vi "TCPIPClienteTeste.vi"() -> ()   [LabVIEW 2012]
uses:
  Setup File/Setup File.lvclass
  RxTXCamera/RxTxCamera.lvclass
  CCDCamera/CCDCamera.lvclass
  CCDCamera/CCDCamera.lvclass/CCDCamera.ctl
  Construct String Setup Cam/Construct String Setup Cam.lvclass
panel:
  in  "Stop":bool
  in  "Start Acquisition":bool
  in  "CCDCamera.lvclass":refnum<class "CCDCamera.lvclass">
  in  "stop":bool
  out "data out":string
  out "Camera Setup":string
  in  "RxTxCamera in":refnum<class "RxTxCamera.lvclass">
  out "Setup 2":T1
  in  "Setup":T1={"Read Mode"="C", "Acquisition Mode"="A", "Trigger"="B", "Exposure Time"="D", "VShift Speed"="E", "Readout rate"="F", "Pre amp"="G", "Shutter Mode"="H", "Shutter TTL"="I", "Time to open shutter"="J", "Time to close shutter"="K", "Cooler"="L", "Temperature"="M", "Initial Line"="N", "Initial Column"="O", "Final Line"="P", "Final Column"="Q", "Horizontal binning"="R", "Vertical binning"="S"}
  in  "Setup File.lvclass":refnum<class "Setup File.lvclass">
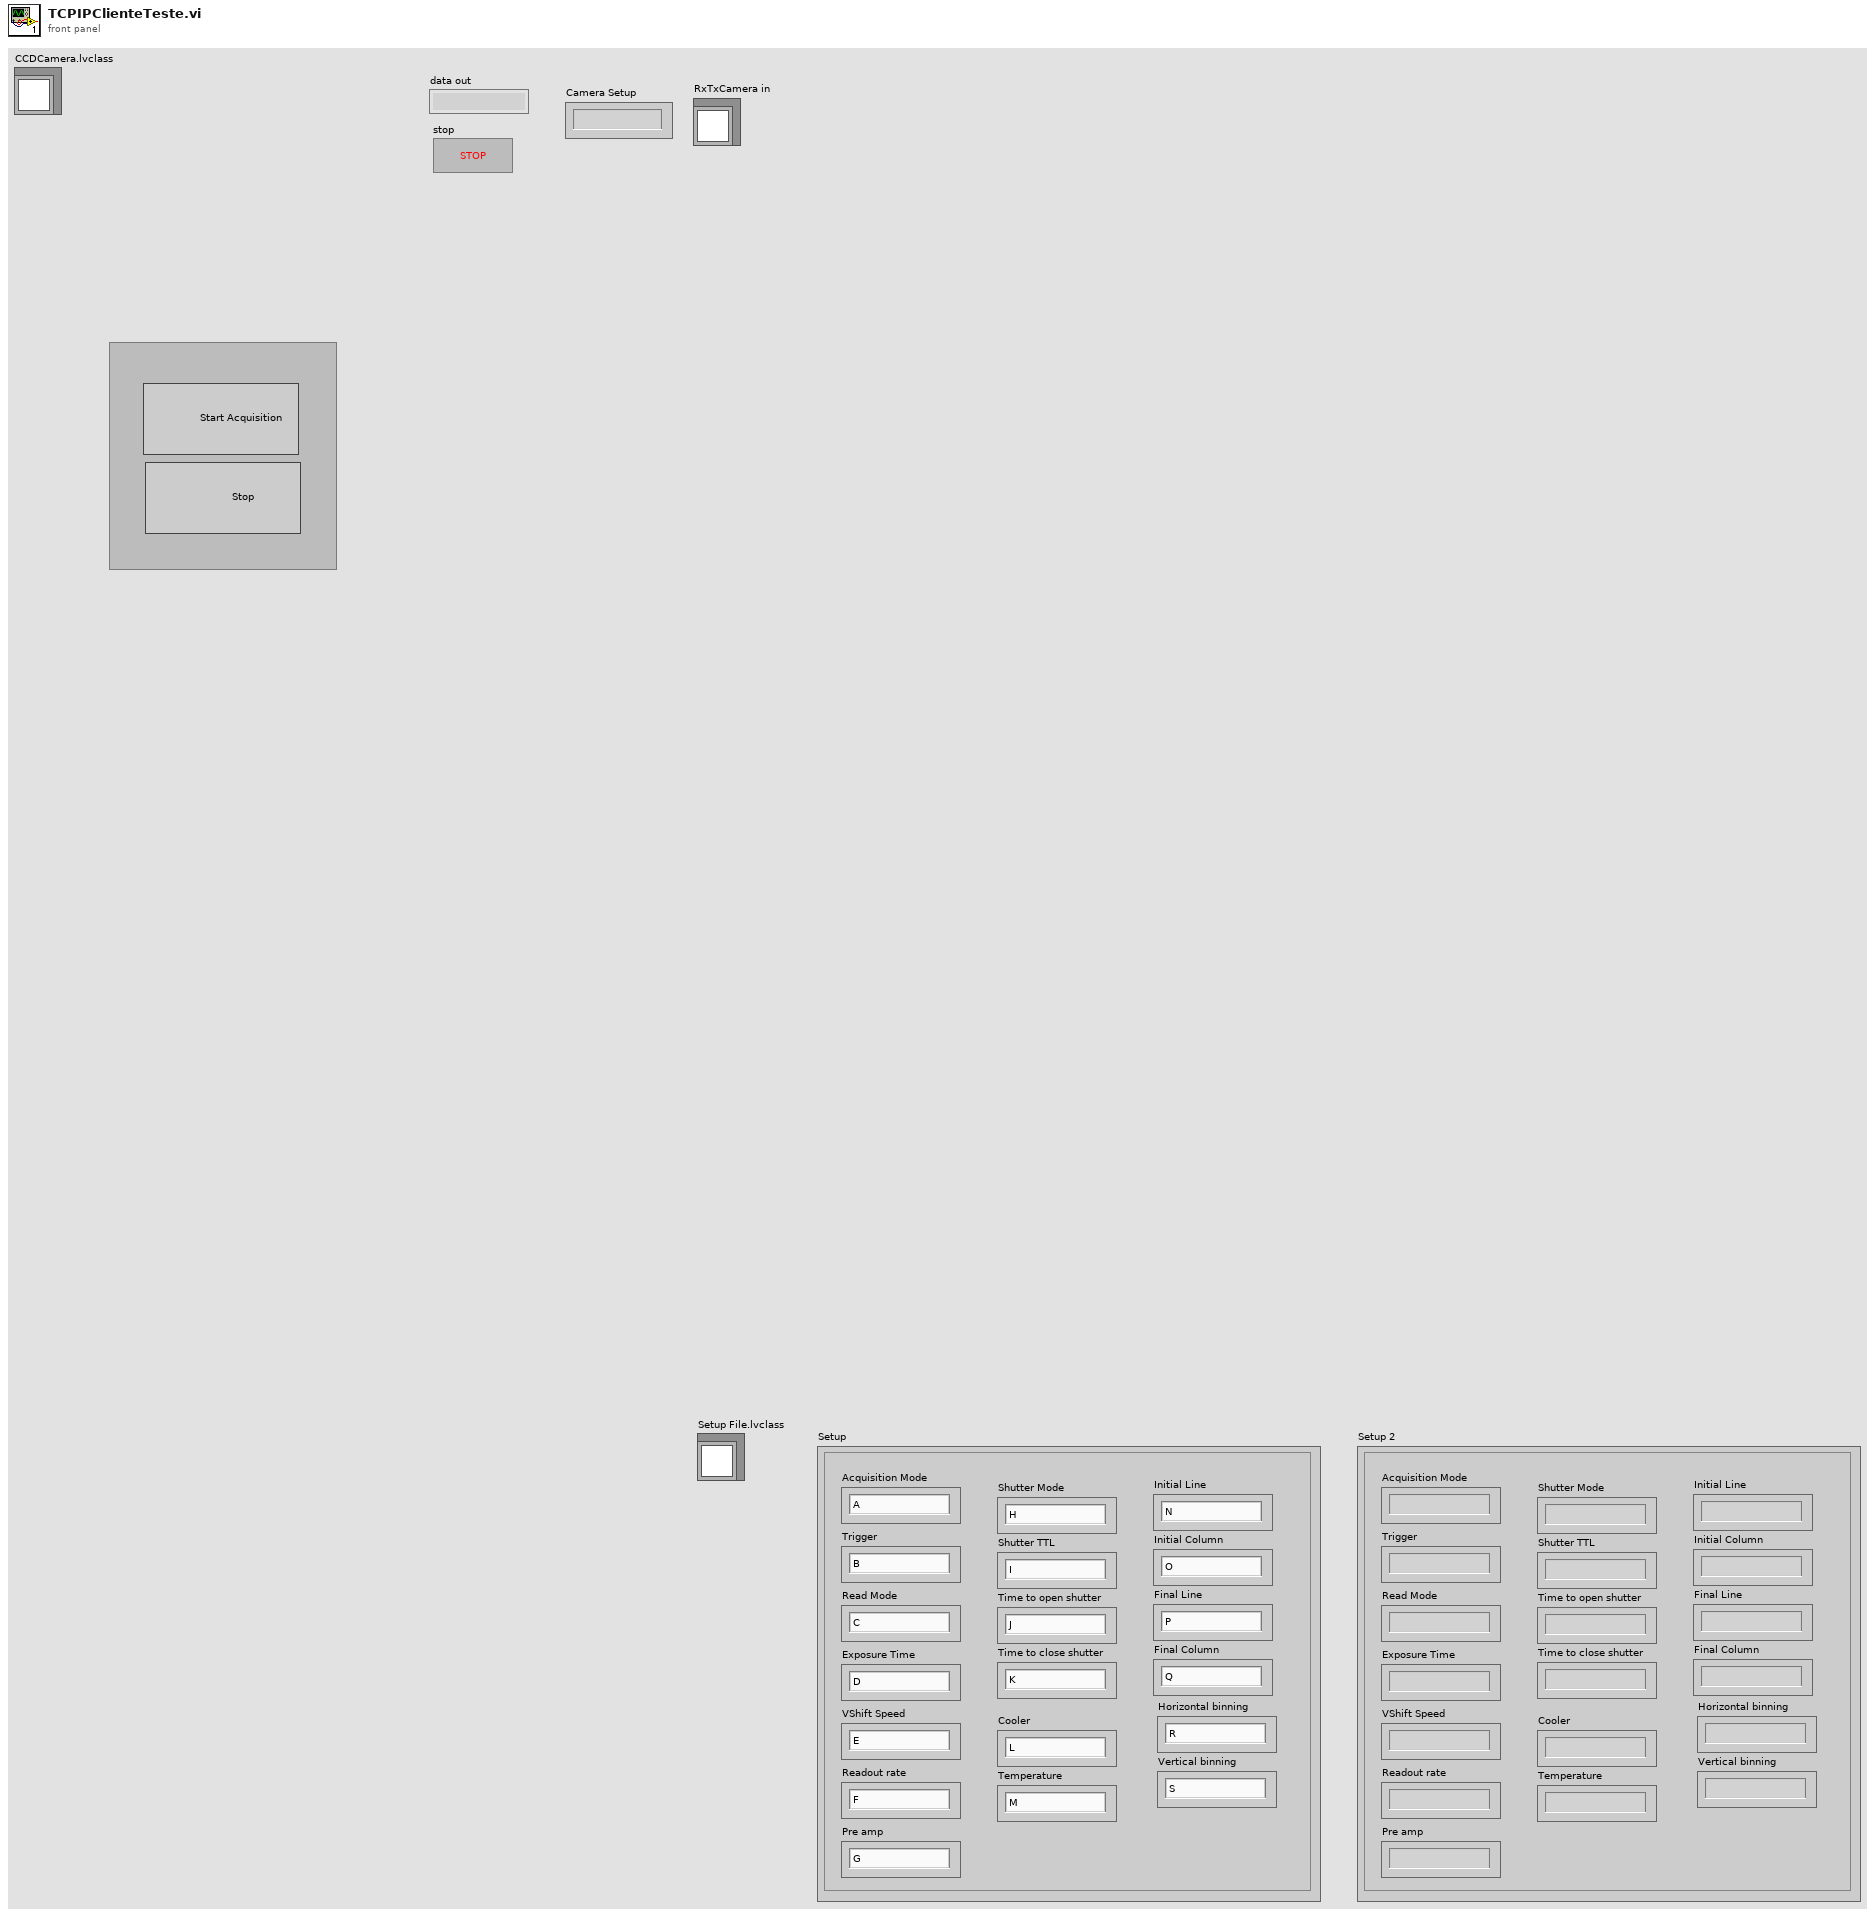
[diagram p1: front panel]
types:
  T1 = cluster{"Read Mode":string, "Acquisition Mode":string, "Trigger":string, "Exposure Time":string, "VShift Speed":string, "Readout rate":string, "Pre amp":string, "Shutter Mode":string, "Shutter TTL":string, "Time to open shutter":string, "Time to close shutter":string, "Cooler":string, "Temperature":string, "Initial Line":string, "Initial Column":string, "Final Line":string, "Final Column":string, "Horizontal binning":string, "Vertical binning":string}
  T2 = cluster{"Read Mode":string, "Acquisition Mode":string, "Trigger":string, "Exposure Time":string, "VShift Speed":string, "Readout rate":string, "Pre amp":string, "Shutter Mode":string, "Shutter TTL":string, "Time to open shutter":string, "Time to close shutter":string, "Cooler":string, "Temperature":string, "Initial Line":string, "Initial Column":string, "Final Line":string, "Final Column":string, "Horizontal binning":string, "Vertical binning":string, "Sub image":string}
  T3 = cluster{"Cooler ON/OFF":u16, "Set temperature":dbl, "Shutter Mode ":u16, "Shutter TTL":u16, "Time to open (ms)":dbl, "Time to close (ms)":dbl, "Pre-amplifier gain":i32, "Vertical clock\n  voltage amplitude":i32, "Vertical Shift Speed":i32, "Readout Rate ":i32, "Trigger ":u16, "Conventional/EM":i32, "Read Mode ":u16, "Acquisition Mode ":u16, "Exposure Time (s) ":sgl, "Initial Line":i32, "Initial Column":i32, "Final Line":i32, "Final Column":i32, "Horizontal binning":i32, "Vertical binning ":i32, "FITS Format":u16, "Image Format":string, "Tiff Position ":u16, "Tiff Type":u16}
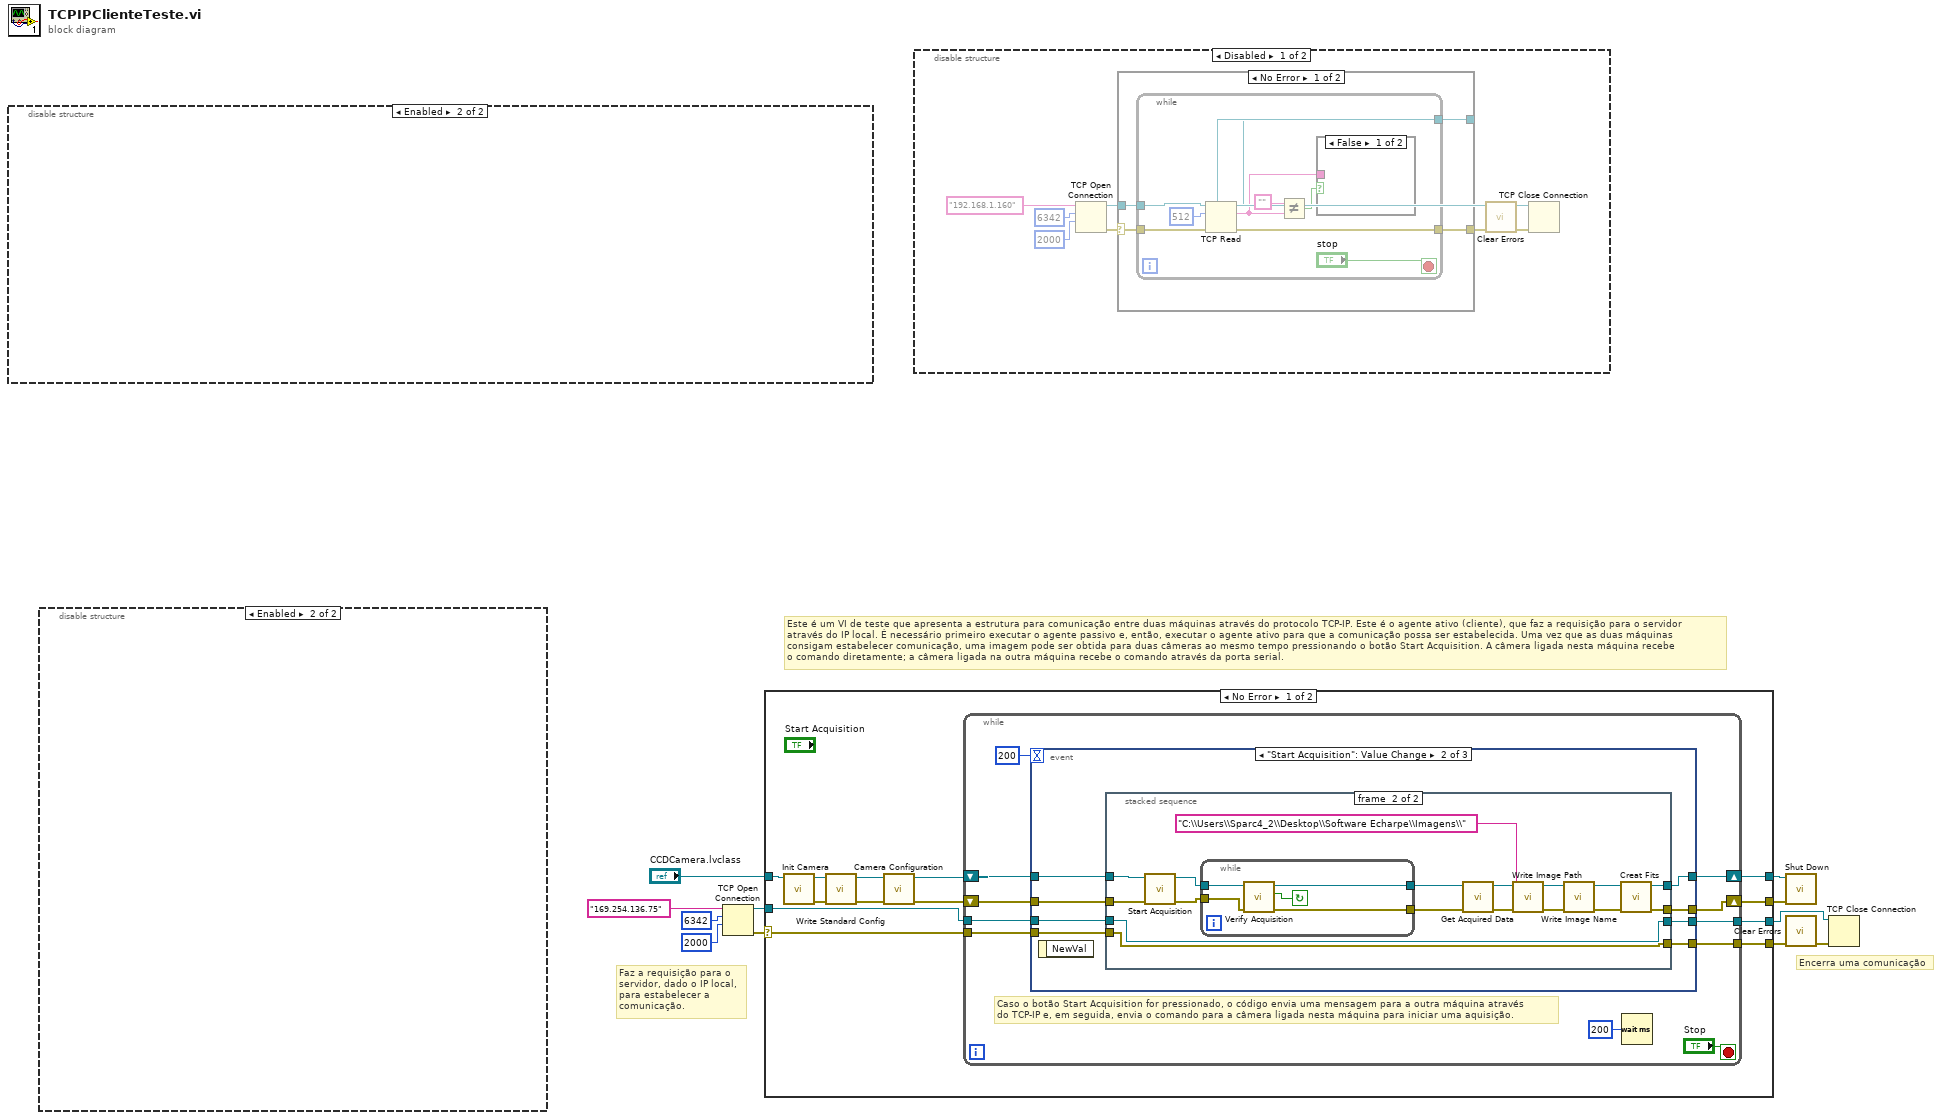
[diagram p0: block diagram]
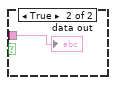
[diagram p2: hidden frame]
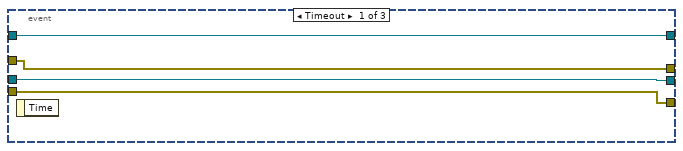
[diagram p5: hidden frame]
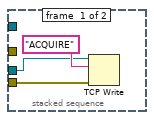
[diagram p6: hidden frame]
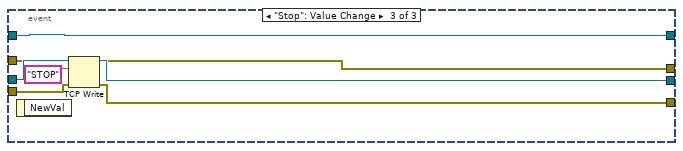
[diagram p7: hidden frame]
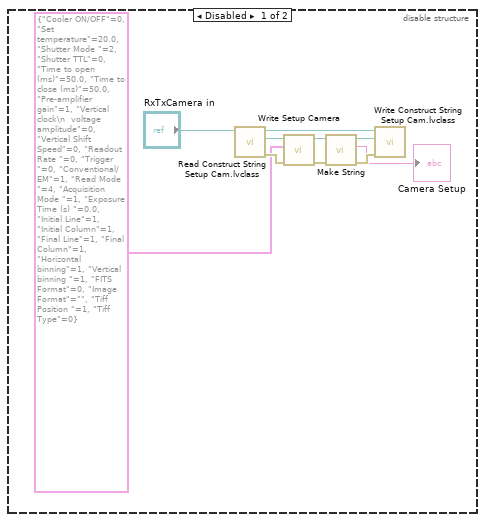
[diagram p9: hidden frame]
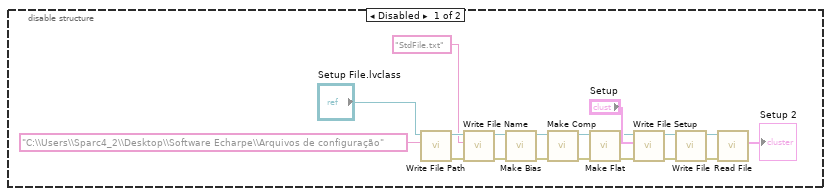
[diagram p10: hidden frame]
diagram:
  # "Encerra uma comunicação"
  # "Faz a requisição para o \nservidor, dado o IP local,\npara estabelecer a \ncomunicação."
  # "Este é um VI de teste que apresenta a estrutura para comunicação entre duas máquinas através do protocolo TCP-IP. Este é o agente ativo (cliente), que faz a requisição para o servidor\natravés do IP local. É necessário primeiro executar o agente passivo e, então, executar o agente ativo para que a comunicação possa ser estabelecida. Uma vez que as duas máquinas\nconsigam estabelecer comunicação, uma imagem pode ser obtida para duas câmeras ao mesmo tempo pressionando o botão Start Acquisition. A câmera ligada nesta máquina recebe \no comando diretamente; a câmera ligada na outra máquina recebe o comando através da porta serial."
  n1 = disable-structure shown="Enabled" {
    frame Disabled {
      n2 = call "Write File Path.vi"("File Path"="C:\\Users\\Sparc4_2\\Desktop\\Software Echarpe\\Arquivos de configuração", "Setup File in"="Setup File.lvclass") -> ("error out"=w28:errorcluster, "Setup File out"=w27:refnum<class "Setup File.lvclass">)  [unwired: 8 in]
      n3 = call "Write File Name.vi"("error in (no error)"=w28, "File Name"="StdFile.txt", "Setup File in"=w27) -> ("error out"=w15:errorcluster, "Setup File out"=w14:refnum<class "Setup File.lvclass">)  [unwired: 7 in]
      n4 = call "Make Bias.vi"("error in (no error)"=w15, "Setup File in"=w14) -> ("error out"=w16:errorcluster, "Setup File out"=w19:refnum<class "Setup File.lvclass">)  [unwired: 8 in]
      n5 = call "Make Comp.vi"("error in (no error)"=w16, "Setup File in"=w19) -> ("error out"=w17:errorcluster, "Setup File out"=w18:refnum<class "Setup File.lvclass">)  [unwired: 8 in]
      n6 = call "Make Flat.vi"("error in (no error)"=w17, "Setup File in"=w18) -> ("error out"=w13:errorcluster, "Setup File out"=w12:refnum<class "Setup File.lvclass">)  [unwired: 8 in]
      n7 = call "Write File Setup.vi"("error in (no error)"=w13, "Setup"="Setup", "Setup File in"=w12) -> ("error out"=w24:errorcluster, "Setup File out"=w23:refnum<class "Setup File.lvclass">)  [unwired: 7 in]
      n8 = call "Write File.vi"("error in (no error)"=w24, "Setup File in"=w23) -> ("error out"=w22:errorcluster, "Setup File out"=w21:refnum<class "Setup File.lvclass">)  [unwired: 8 in]
      n9 = call "Read File.vi"("error in (no error)"=w22, "Setup File in"=w21) -> ("Setup"=→"Setup 2":T2)  [unwired: 7 in, 2 out]
    }
    frame Enabled {
    }
  }
  n10 = disable-structure shown="Enabled" {
    frame Disabled {
      n11 = call "Read Construct String Setup Cam.lvclass.vi"("RxTxCamera in"="RxTxCamera in") -> ("error out"=w34:errorcluster, "Construct String Setup Cam.lvclass"=w37:refnum<class "Construct String Setup Cam.lvclass">, "RxTxCamera out"=w35:refnum<class "RxTxCamera.lvclass">)  [unwired: 8 in]
      n12 = call "Write Setup Camera.vi"("error in (no error)"=w34, "RED Channel Settings"=T3 {"Cooler ON/OFF"=0, "Set temperature"=20.0, "Shutter Mode "=2, "Shutter TTL"=0, "Time to open (ms)"=50.0, "Time to close (ms)"=50.0, "Pre-amplifier gain"=1, "Vertical clock\n  voltage amplitude"=0, "Vertical Shift Speed"=0, "Readout Rate "=0, "Trigger "=0, "Conventional/EM"=1, "Read Mode "=4, "Acquisition Mode "=1, "Exposure Time (s) "=0.0, "Initial Line"=1, "Initial Column"=1, "Final Line"=1, "Final Column"=1, "Horizontal binning"=1, "Vertical binning "=1, "FITS Format"=0, "Image Format"="", "Tiff Position "=1, "Tiff Type"=0}, "Construct String Setup Cam in"=w37) -> ("error out"=w40:errorcluster, "Construct String Setup Cam out"=w39:refnum<class "Construct String Setup Cam.lvclass">)  [unwired: 7 in]
      n13 = call "Make String.vi"("error in (no error)"=w40, "Construct String Setup Cam in"=w39) -> ("error out"=w33:errorcluster, "Camera Setup"=→"Camera Setup":string, "Construct String Setup Cam out"=w36:refnum<class "Construct String Setup Cam.lvclass">)  [unwired: 7 in]
      n14 = call "Write Construct String Setup Cam.lvclass.vi"("error in (no error)"=w33, "Construct String Setup Cam.lvclass"=w36, "RxTxCamera in"=w35) -> ()  [unwired: 7 in, 2 out]
    }
    frame Enabled {
    }
  }
  n15 = TCP Open Connection(address="169.254.136.75", remote port or service name=u16 6342, timeout ms (60000)=2000) -> (connection ID=w4:refnum<k5>, error out=w8:errorcluster)  [unwired: 2 in]
  n16 = case shown="No Error" w8 {
    selector: w8 -> [w53 w109]
    tunnel: [w50 _] -> w7
    tunnel: [w51 w111] -> w6
    tunnel: "CCDCamera.lvclass" -> [w47 w111]
    tunnel: w4 -> [w52 w110]
    tunnel: [w46 w110] -> w2
    tunnel: [w45 w109] -> w1
    frame No Error {
      n17 = call "Init Camera.vi"("CCDCamera in"=w47) -> ("error out"=w48:errorcluster, "CCDCamera out"=w49:refnum<class "CCDCamera.lvclass">)  [unwired: 9 in]
      n18 = call "Write Standard Config.vi"("error in (no error)"=w48, "CCDCamera in"=w49) -> ("error out"=w44:errorcluster, "CCDCamera out"=w41:refnum<class "CCDCamera.lvclass">)  [unwired: 8 in]
      n19 = call "Camera Configuration.vi"("error in (no error)"=w44, "CCDCamera in"=w41) -> ("error out"=w43:errorcluster, "CCDCamera out"=w42:refnum<class "CCDCamera.lvclass">)  [unwired: 8 in]
      n20 = while {
        tunnel: w53 -> [w61]
        tunnel: w52 -> [w60]
        shift-right: [w59] -> w51
        shift-left: w42 -> [w62]
        shift-right: [w58] -> w50
        shift-left: w43 -> [w57]
        tunnel: [w56] -> w46
        tunnel: [w55] -> w45
        stop <- "Stop" stop-if-true
        # "Caso o botão Start Acquisition for pressionado, o código envia uma mensagem para a outra máquina através\ndo TCP-IP e, em seguida, envia o comando para a câmera ligada nesta máquina para iniciar uma aquisição."
        n21 = event shown="[1] \"Start Acquisition\": Value Change" {
          selector: _ -> [_ _ _]
          dyn-events: _ -> [_ _ _]
          timeout: 200 -> [_ _ _]
          tunnel: w62 -> [w68 w76 w102]
          tunnel: w61 -> [w66 w75 w108]
          tunnel: w60 -> [w67 w74 w107]
          tunnel: [w68 w73 w102] -> w59
          tunnel: [w65 w72 w103] -> w58
          tunnel: w57 -> [w65 w71 w103]
          tunnel: [w67 w70 w105] -> w56
          tunnel: [w66 w69 w104] -> w55
          event Timeout {
            n22 = event-data() -> ()  [unwired: 1 in, 1 out]
          }
          event "Start Acquisition": Value Change {
            n23 = event-data() -> ()  [unwired: 1 in, 1 out]
            n24 = stacked-sequence {
              tunnel: w76 -> [_ w90]
              tunnel: w75 -> [w78 w88]
              tunnel: w74 -> [w77 w89]
              tunnel: [_ w93] -> w73
              tunnel: [_ w92] -> w72
              tunnel: w71 -> [_ w91]
              tunnel: [_ w89] -> w70
              tunnel: [_ w88] -> w69
              frame #0 {
                n25 = TCP Write(connection ID=w77, data in="ACQUIRE", error in (no error)=w78) -> ()  [unwired: 1 in, 3 out]
              }
              frame #1 {
                n26 = call "Start Acquisition.vi"("error in (no error)"=w91, "CCDCamera in"=w90) -> ("error out"=w96:errorcluster, "CCDCamera out"=w95:refnum<class "CCDCamera.lvclass">)  [unwired: 8 in]
                n27 = while {
                  tunnel: w96 -> [w101]
                  tunnel: [w100] -> w87
                  tunnel: [w99] -> w86
                  tunnel: w95 -> [w98]
                  stop <- w97 continue-if-true
                  n28 = call "Verify Acquisition.vi"("error in (no error)"=w101, "CCDCamera in"=w98) -> ("error out"=w100:errorcluster, "Acquiring"=w97:bool, "CCDCamera out"=w99:refnum<class "CCDCamera.lvclass">)  [unwired: 7 in]
                }
                n29 = call "Get Acquired Data.vi"("error in (no error)"=w87, "CCDCamera in"=w86) -> ("error out"=w84:errorcluster, "CCDCamera out"=w85:refnum<class "CCDCamera.lvclass">)  [unwired: 8 in]
                n30 = call "Write Image Path.vi"("error in (no error)"=w84, "Image Path"="C:\\Users\\Sparc4_2\\Desktop\\Software Echarpe\\Imagens\\", "CCDCamera in"=w85) -> ("error out"=w83:errorcluster, "CCDCamera out"=w80:refnum<class "CCDCamera.lvclass">)  [unwired: 7 in]
                n31 = call "Write Image Name.vi"("error in (no error)"=w83, "CCDCamera in"=w80) -> ("error out"=w82:errorcluster, "CCDCamera out"=w81:refnum<class "CCDCamera.lvclass">)  [unwired: 8 in]
                n32 = call "Creat Fits.vi"("error in (no error)"=w82, "CCDCamera in"=w81) -> ("error out"=w92:errorcluster, "CCDCamera out"=w93:refnum<class "CCDCamera.lvclass">)  [unwired: 8 in]
              }
            }
          }
          event "Stop": Value Change {
            n33 = event-data() -> ()  [unwired: 1 in, 1 out]
            n34 = TCP Write(connection ID=w107, data in="STOP", error in (no error)=w108) -> (connection ID out=w105:refnum<k5>, error out=w104:errorcluster)  [unwired: 1 in, 1 out]
          }
        }
        n35 = Wait (ms)(milliseconds to wait=u32 200) -> ()  [unwired: 1 out]
      }
    }
    frame Error {
    }
  }
  n36 = disable-structure shown="Disabled" {
    frame Disabled {
      n37 = TCP Open Connection(address="192.168.1.160", remote port or service name=u16 6342, timeout ms (60000)=2000) -> (connection ID=w117:refnum<k5>, error out=w118:errorcluster)  [unwired: 2 in]
      n38 = case shown="No Error" w118 {
        selector: w118 -> [w122 w134]
        tunnel: w117 -> [w123 w135]
        tunnel: [w121 w134] -> w113
        tunnel: [w120 w135] -> w116
        frame No Error {
          n39 = while {
            tunnel: w123 -> [w132]
            tunnel: w122 -> [w131]
            tunnel: [w130] -> w121
            tunnel: [w129] -> w120
            stop <- "stop" stop-if-true
            n40 = TCP Read(connection ID=w132, bytes to read=512, error in (no error)=w131) -> (connection ID out=w129:refnum<k5>, data out=w126:string, error out=w130:errorcluster)  [unwired: 2 in]
            n41 = Not Equal?(x="", y=w126) -> (x != y?=w127:bool)
            n42 = case shown="False" w127 {
              tunnel: w126 -> [_ w133]
              frame False {
              }
              frame True {
                "data out" <- w133
              }
            }
          }
        }
        frame Error {
        }
      }
      n43 = call <vilib>:"Clear Errors.vi"("error in (no error)"=w113) -> ("error out"=w112:errorcluster)  [unwired: 6 in]
      n44 = TCP Close Connection(connection ID=w116, error in (no error)=w112) -> ()  [unwired: 1 in, 2 out]
    }
    frame Enabled {
    }
  }
  n45 = call "Shut Down.vi"("error in (no error)"=w7, "CCDCamera in"=w6) -> ()  [unwired: 8 in, 2 out]
  n46 = call <vilib>:"Clear Errors.vi"("error in (no error)"=w1) -> ("error out"=w3:errorcluster)  [unwired: 6 in]
  n47 = TCP Close Connection(connection ID=w2, error in (no error)=w3) -> ()  [unwired: 1 in, 2 out]
